vi "Test Check Dirty.vi"() -> ()   [LabVIEW 2020, in "GPack.lvlib" / "GitPackage.lvclass"]
uses:
  GitPackage.lvclass
  GitPackage.lvclass/GitPackage.ctl
panel:
  out "Dirty":bool
  in  "Folder":path=path "C:/dev/lv20CE/relink/lv-cdm"
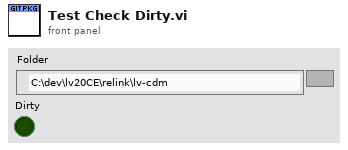
[diagram p1: front panel]
types:
  T1 = typedef "GPack.lvlib/Package Info.ctl" = cluster{"Name":string, "Type":string, "Host":string, "Path":string, "Branch":string, "Version":string}
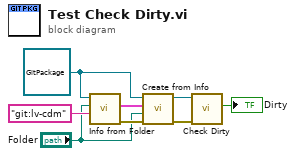
[diagram p0: block diagram]
diagram:
  w5 = refnum<class "GitPackage.lvclass"> refnum ("GPack.lvlib:GitPackage.lvclass")
  n1 = call-dynamic "Info from Folder.vi"("Name"="git:lv-cdm", "Folder"="Folder", "GitPackage in"=w5) -> ("error out"=w8:errorcluster, "Package Info"=w6:T1)  [unwired: 7 in]
  n2 = call-dynamic "Create from Info.vi"("error in (no error)"=w8, "Folder"="Folder", "Package Info"=w6, "GitPackageAbstract in"=w5) -> ("error out"=w2:errorcluster, "GitPackageAbstract out"=w3:refnum<class "GitPackage.lvclass">)  [unwired: 6 in]
  n3 = call-dynamic "Check Dirty.vi"("error in (no error)"=w2, "GitPackage in"=w3) -> ("Dirty"=→"Dirty":bool)  [unwired: 7 in, 2 out]
